vi "EBARA_Timer.vi"(1 "Time Intv":u32) -> (0 "N2 Valve":bool)   [LabVIEW 2011]
uses:
  DynaGlbs.vi
  SysGlbs.vi
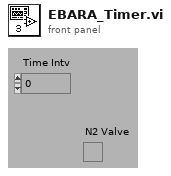
[diagram p1: front panel]
types:
  T1 = cluster{"Press":u8[], "PD_cell":cluster{"H2_cell":u8, "H2_line":u8, "horn":u8, "light":u8, "temp":u8, "PD_cell?":bool, "Temp Set":u16, "N2_in":u8, "N2_line":u8}, "RampDn":u8[], "GV/LL":cluster{"LL Door":u8, "GV Up":u8, "GV Low":u8, "GV _LIn":u8, "Fork":u8, "GV_UIn":u8, "GC Press":u8, "LL Press":u8, "MDA_LL":u8[], "Motor":u8, "EQ Valve":u8, "LL Active":u8}, "GC_Pump":cluster{"LL_Vac":u8, "GC_Vac":u8, "Bypass":u8, "Rough":u8, "Isolat":u8, "LL_MDA":u8[], "Vac_Press":u8, "TGV":u8}, "N2 Purge":cluster{"N2_LL":u8, "MFC":u8}, "RampRate":dbl[], "GC_Vac":cluster{"D_Vac-":u8[], "D_Vac+":u8[], "A_Vac":u8[], "D_Open+":u8[], "D_Open-":u8[], "A_Open":u8[]}, "Toxic":u8[], "Indicators":u8[], "LL Routine":cluster{"D Open":u8[], "D Close":u8[], "Timeout(ms)":u32}, "Temperature":u8[], "EBARA Pump":cluster{"EBARA_Din":cluster{"Main Status":u8, "Booster Status":u8, "Indicator":u8, "N2 Isolat":u8}, "EBARA_N2":u8[]}}
  T2 = cluster{"Main Status":u8, "Booster Status":u8, "Indicator":u8, "N2 Isolat":u8}
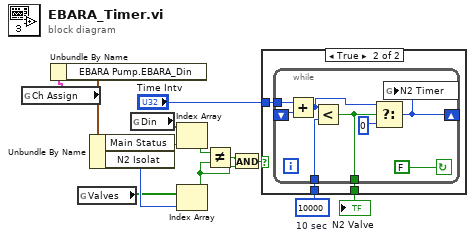
[diagram p0: block diagram]
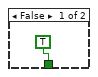
[diagram p2: hidden frame]
diagram:
  w7 = 10000  # 10 sec
  n1 = global read "SysGlbs.vi" "Ch Assign"() -> (w2:T1)
  n2 = Unbundle By Name(w2) -> ("EBARA Pump.EBARA_Din"=w1:T2)
  n3 = global read "DynaGlbs.vi" "Valves"() -> (w10:bool[])
  n4 = Unbundle By Name(w1) -> ("Main Status"=w13:u8, "N2 Isolat"=w11:u8)
  n5 = global read "DynaGlbs.vi" "Din"() -> (w12:bool[])
  n6 = Index Array(array=w12, index=w13) -> (element=w9:bool)
  n7 = Index Array(array=w10, index=w11) -> (element=w4:bool)
  n8 = Not Equal?(x=w9, y=w4) -> (x != y?=w5:bool)
  n9 = And(x=w5, y=w4) -> (x .and. y?=w3:bool)
  n10 = case shown="True" w3 {
    tunnel: "Time Intv" -> [_ w17]
    tunnel: w7 -> [_ w16]
    tunnel: [TRUE w15] -> w6
    frame False {
    }
    frame True {
      n11 = while {
        shift-right: [w19] -> _
        shift-left: _ -> [w24]
        tunnel: w17 -> [w25]
        tunnel: w16 -> [w23]
        tunnel: [w20] -> w15
        stop <- FALSE continue-if-true
        n12 = Add(x=w25, y=w24) -> (x+y=w22:u32)
        n13 = Less?(x=w22, y=w23) -> (x < y?=w20:bool)
        n14 = Select(t=w22, s=w20, f=0) -> (s? t:f=w19:u32)
        n15 = global write "DynaGlbs.vi" "N2 Timer"(w19) -> ()
      }
    }
  }
  "N2 Valve" <- w6
